vi "Update Calibration Samples and Selection.vi"(7 "N-Samples":i32, 8 "error in (no error)":errorcluster, 9 "Selection":i32, 10 "Sample":T1, 11 "UI in":refnum<class "UI.lvclass">) -> (0 "error out":errorcluster)   [LabVIEW 2020, in "AR Example.lvlib" / "UI.lvclass"]
uses:
  UI.lvclass
  g_ar_toolkit.image/ARGB Image.ctl
  UI.lvclass/UI.ctl
  g_ar_toolkit.image/Size (ARGB).vi
  g_ar_toolkit.image/Draw Image to Picture (ARGB).vi
  g_ar_toolkit.image/Size (ARGB).vi/69a1505b-b287-44ed-9ef9-f10ed7b260f4.vi
  g_ar_toolkit.image/Draw Image to Picture (ARGB).vi/8cd07b1b-062e-4fe4-9e87-2eb3dc89fe0e.vi
  g_ar_toolkit.common/Module Path.vi
  <vilib>/Utility/error.llb/Error Cluster From Error Code.vi
  g_ar_toolkit.image/g_ar_toolkit.image.lvlib
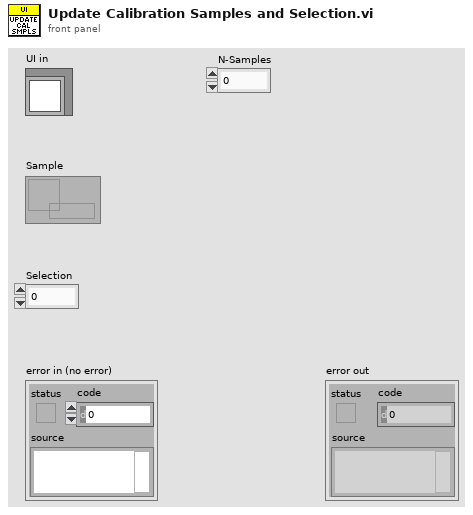
[diagram p1: front panel]
types:
  T1 = typedef "g_ar_toolkit.image.lvlib/ARGB Image.ctl" = refnum<data-value>
  T2 = cluster{"Remove":bool, "Left":bool, "Right":bool}
  T3 = typedef "g_ar_toolkit.common.lvlib/Image Size (Integer).ctl" = cluster{"Width":u16, "Height":u16}
  T4 = typedef "g_ar_toolkit.image.lvlib/Image Draw Offset.ctl" = cluster{"Left":i16, "Top":i16}
  T5 = enum8{"Enabled", "Disabled", "Disabled and Grayed Out"}
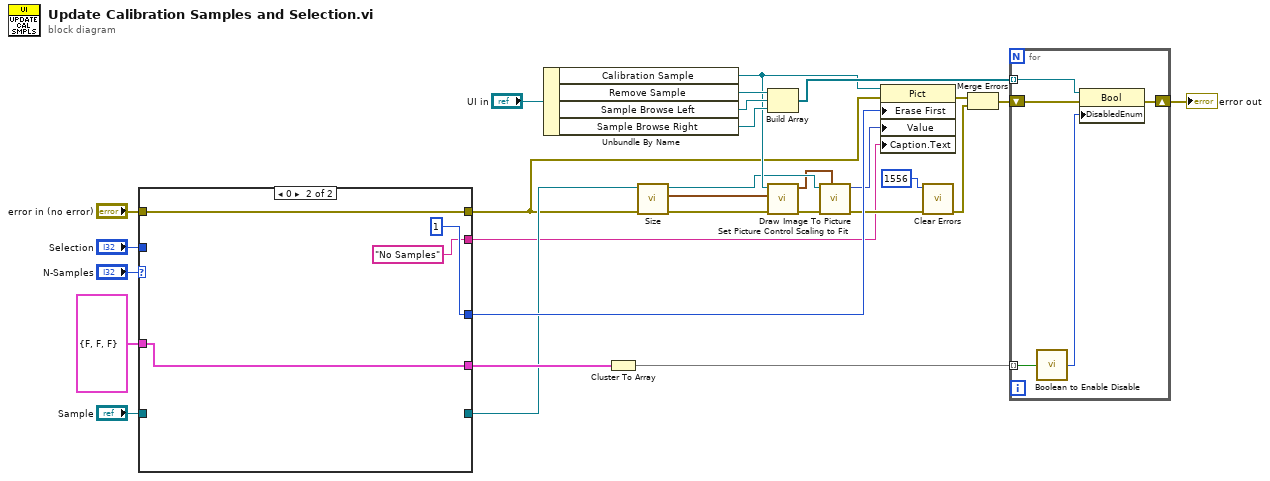
[diagram p0: block diagram]
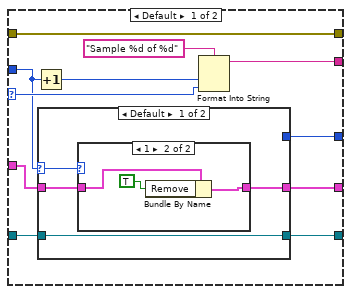
[diagram p2: hidden frame]
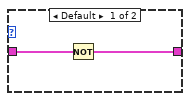
[diagram p3: hidden frame]
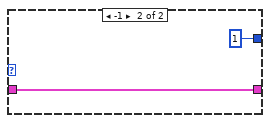
[diagram p4: hidden frame]
diagram:
  n1 = case shown="0" "N-Samples" {
    selector: "N-Samples" -> [w31 _]
    tunnel: "error in (no error)" -> [w35 w55]
    tunnel: [w35 w55] -> w13
    tunnel: [w38 u8 1 ("unsigned 8bit integer")] -> w27
    tunnel: "Selection" -> [w30 _]
    tunnel: T2 {"Remove"=FALSE, "Left"=FALSE, "Right"=FALSE} -> [w39 w54]
    tunnel: [w40 w54] -> w21
    tunnel: "Sample" -> [w37 _]
    tunnel: [w36 _] -> w16
    tunnel: [w32 "No Samples"] -> w1
    frame Default {
      n2 = Increment(x=w30) -> (x+1=w34:i32)
      n3 = case shown="Default" w30 {
        selector: w30 -> [w44 _]
        tunnel: [w42 w51] -> w40
        tunnel: w39 -> [w43 w51]
        tunnel: [_ u8 1] -> w38
        tunnel: w37 -> [w41 _]
        tunnel: [w41 _] -> w36
        frame Default {
          n4 = case shown="1" w44 {
            tunnel: w43 -> [w46 w49]
            tunnel: [w45 w48] -> w42
            frame Default {
              n5 = Not(x=w46) -> (.not. x?=w45:T2)
            }
            frame 1 {
              n6 = Bundle By Name(cluster=w49, "Remove"=TRUE) -> (w48:T2)
            }
          }
        }
        frame -1 {
        }
      }
      n7 = Format Into String(format string="Sample %d of %d", w34, w31) -> (resulting string=w32:string)  [unwired: 2 in, 1 out]
    }
    frame 0 {
    }
  }
  n8 = Unbundle By Name("UI in") -> ("Calibration Sample"=w14:refnum<vi>, "Remove Sample"=w26:refnum<vi>, "Sample Browse Left"=w24:refnum<vi>, "Sample Browse Right"=w23:refnum<vi>)
  n9 = Cluster To Array(cluster=w21) -> (array=w20:bool[])
  n10 = call-poly "Size.vi"("error in (no error)"=w13, "ARGB Image"=w16) -> ("error out"=w12:errorcluster, "Image Size"=w15:T3, "ARGB Image (duplicate)"=w10:T1)  [unwired: 7 in]
  n11 = Build Array(w26, w24, w23) -> (w22:refnum<vi>[])
  n12 = call "Set Picture Control Scaling to Fit.vi"("error in (no error)"=w12, "Image Size"=w15, "Picture in"=w14) -> ("error out"=w11:errorcluster, "Image Draw Offset"=w9:T4)  [unwired: 7 in]
  n13 = call-poly "Draw Image To Picture.vi"("Image Draw Offset (Default 0,0)"=w9, "error in (no error)"=w11, "ARGB Image Source"=w10) -> ("error out"=w7:errorcluster, "Picture"=w8:picture)  [unwired: 7 in]
  n14 = property class="Pict"(reference=w14, error in=w13, "Erase First"=w27, "Value"=w8, "Caption.Text"=w1) -> (error out=w18:errorcluster)  [unwired: 1 out]
  n15 = call <vilib>:"Clear Errors.vi"("error in (no error)"=w7, "specific error code to clear (0: all)"=1556) -> ("error out"=w4:errorcluster)  [unwired: 4 in, 1 out]
  n16 = Merge Errors(w18, w4) -> (w5:errorcluster)
  n17 = for {
    tunnel: w22 -> [w60] mode=indexing
    tunnel: w20 -> [w59] mode=indexing
    shift-right: [w56] -> w17
    shift-left: w5 -> [w57]
    n18 = call "Boolean to Enable Disable.vi"("Enable?"=w59) -> ("Enable/Disable"=w58:T5)
    n19 = property class="Bool"(reference=w60, error in=w57, "DisabledEnum"=w58) -> (error out=w56:errorcluster)  [unwired: 1 out]
  }
  "error out" <- w17
